vi "Fit Logistic Square Pulse.vi"(0 "Decay":T14, 1 "Optimal Offset Selection Criterion":T1, 5 "Boundaries":dbl[](array[numeric]), 9 "Basic Fit Options":T4, 11 "error in (no error)":errorcluster, 12 "Square Pulse Options":T2={"Method"=enum."Mode", "# Bins"=0, "Threshold %"=10.0, "Center on Midpoint"=TRUE, "Smoothen Plot"=FALSE}) -> (4 "Fitted Decay":cluster{"t Array":dbl[], "Fitted Array":dbl[]}, 6 "Residuals":cluster{"t Array":dbl[], "Residual Array":dbl[]}, 8 "Fit Output":T9={"best nonlinear fit"=[], "best fit parameters"=[], "R^2"=0.0, "RMSE"=0.0, "error out"={"status"=FALSE, "code"=0, "source"=""}, "Fitting Method"=enum."Least Square", "number of function calls"=0, "number of iterations"=0, "covariance"=[], "Chi 2"=0.0, "DOF"=0, "Fit Convergence Criterion"=enum."Continue", "Fitting Algorithm"=enum."Levenberg-Marquardt", "Weighted Fit"=enum."Unweighted", "Gradient"=0.0, "|Delta Chi 2|"=0.0, "|Delta Chi 2|/Chi 2"=0.0, "Max |Delta a| /|a|"=0.0, "Lambda"=-1.0, "RSS"=0.0, "AIC"=0.0, "BIC"=0.0, "Max number of function calls"=0, "Max number of iterations"=0, "IRF"={"X Array"=[], "Y Array"=[]}, "IRF Normalization Factor"=0.0, "Decay Normalization Factor"=0.0, "Number of offset fits"=0, "Weighted Chi2"=-1.0, "Unweighted Chi2"=-1.0}, 10 "Delta Best Fit Parameters":dbl[](array[numeric]), 15 "error out":errorcluster)   [LabVIEW 2021, in "Fits.lvlib"]
uses:
  Fits.lvlib
  ee5d1f48-236f-4ce4-8b82-c8db8954dd38.vi
  Time/Time.lvlib
  <vilib>/ErrorRing/Error Ring.xnode
  <vilib>/Utility/error.llb/DialogType.ctl
  LM model Function and gradient (Logistic Square-Gated IRF).vi
  <vilib>/Utility/error.llb/Error Cluster From Error Code.vi
  Arrays/Arrays.lvlib
  Graphs/XY Graph/XY Graph Plot Data.ctl
  Graphs/XY Graph/XY Graph Add-Ons.lvlib
  Decay Convolution/Fit Control Data.ctl
  <vilib>/Analysis/Matrix/Datatypes/RealMatrix.ctl
  <vilib>/Analysis/Matrix/NI_Matrix.lvlib
  Non-linear Fit Output v4.ctl
  Residual Type.ctl
  Basic Fit Options.ctl
  Square Pulse Levels Type.ctl
  Square Pulse Options.ctl
  Convergence Criteria.ctl
  Non-linear Fitting Algorithm.ctl
  Non-linear Fitting Method v2.ctl
  Nonlinear Fit Method.ctl
  Optimal Offset Selection Criterion.ctl
  IRF(X)PSED/Fit Weights Type v2.ctl
panel:
  out "XY Graph":cluster{"X Array":dbl[], "Y Array":dbl[]}[](graph)
  out "CPU (s)":dbl
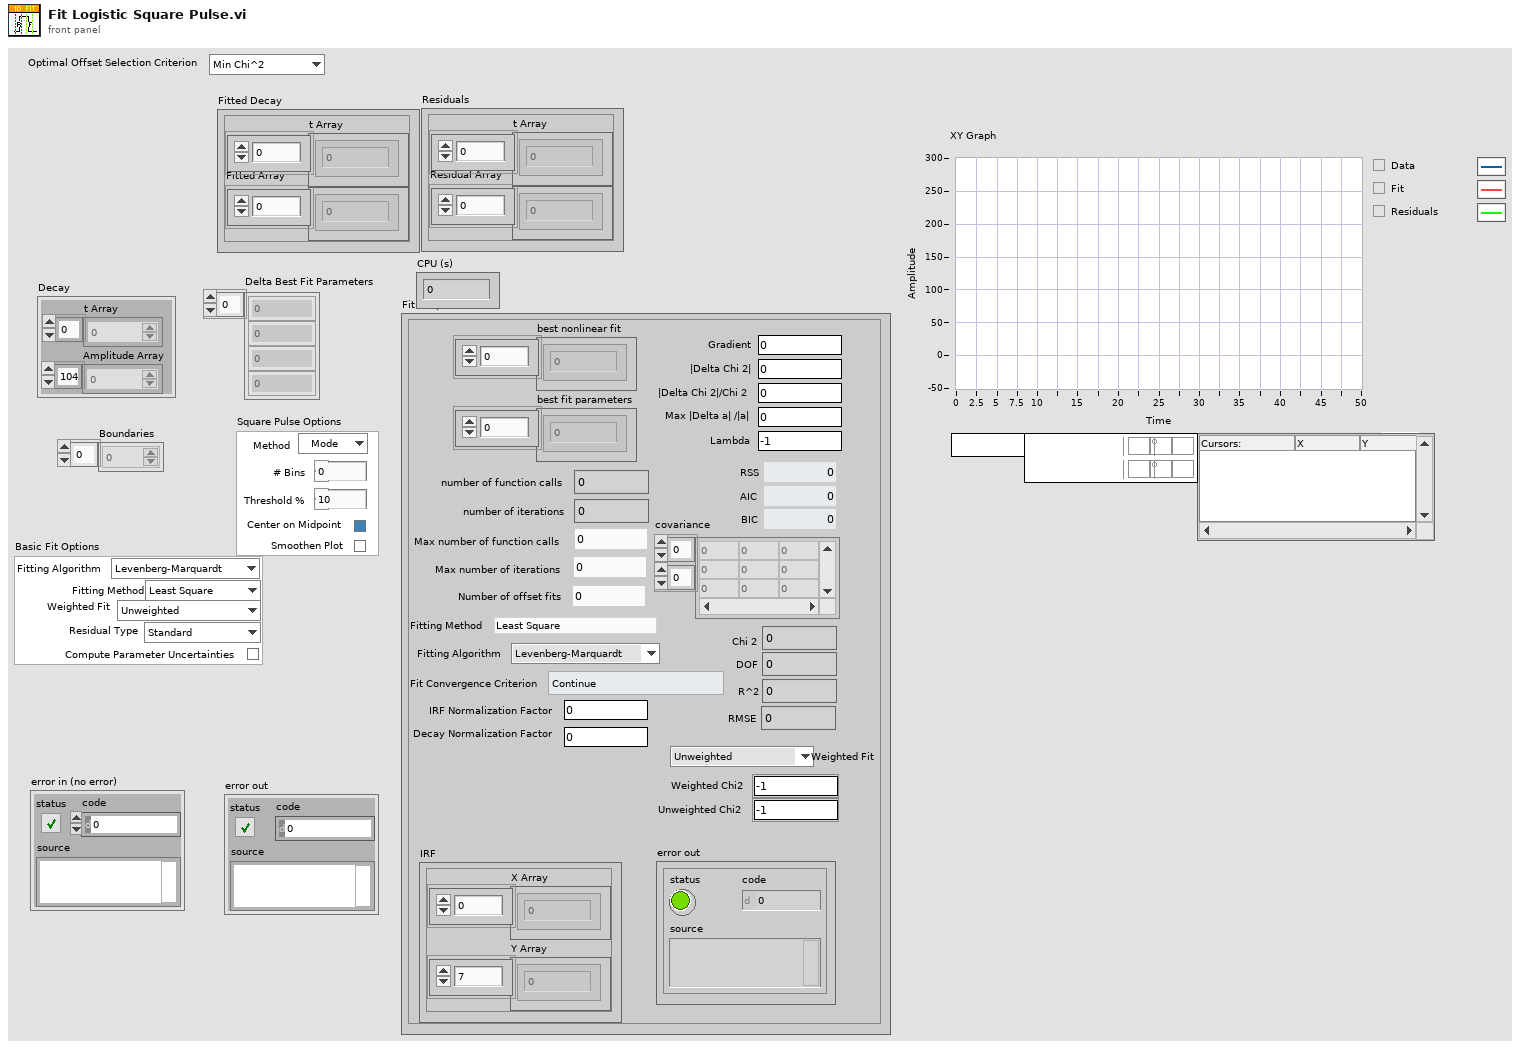
[diagram p1: front panel]
types:
  T1 = typedef "Fits.lvlib/Optimal Offset Selection Criterion.ctl" = enum16{"Min Chi^2", "Max R^2"}
  T2 = typedef "Fits.lvlib/Square Pulse Options.ctl" = cluster{"Method":T3, "# Bins":i32, "Threshold %":dbl, "Center on Midpoint":bool, "Smoothen Plot":bool}
  T3 = typedef "Fits.lvlib/Square Pulse Levels Type.ctl" = enum16{"Mode", "Mean"}
  T4 = typedef "Fits.lvlib/Basic Fit Options.ctl" = cluster{"Fitting Method":T5, "Weighted Fit":T6, "Residual Type":T7, "Compute Parameter Uncertainties":bool, "Fitting Algorithm":T8}
  T5 = typedef "Fits.lvlib/Non-linear Fitting Method v2.ctl" = enum16{"Least Square", "Least Absolute Residual", "Bisquare", "MLE", "-", "Best of All"}
  T6 = typedef "Fits.lvlib/Fit Weights Type v2.ctl" = enum16{"Unweighted", "1/Variance (Neyman)", "1/Variance (Pearson)", "Best of All"}
  T7 = typedef "Fits.lvlib/Residual Type.ctl" = enum16{"Standard", "Normalized", "Reduced"}
  T8 = typedef "Fits.lvlib/Non-linear Fitting Algorithm.ctl" = enum16{"Levenberg-Marquardt", "Trust-Region Dogleg"}
  T9 = typedef "Fits.lvlib/Non-linear Fit Output v4.ctl" = cluster{"best nonlinear fit":dbl[], "best fit parameters":dbl[], "R^2":dbl, "RMSE":dbl, "error out":errorcluster, "Fitting Method":T10, "number of function calls":i32, "number of iterations":i32, "covariance":T11, "Chi 2":dbl, "DOF":i32, "Fit Convergence Criterion":T12, "Fitting Algorithm":T8, "Weighted Fit":T6, "Gradient":dbl, "|Delta Chi 2|":dbl, "|Delta Chi 2|/Chi 2":dbl, "Max |Delta a| /|a|":dbl, "Lambda":dbl, "RSS":dbl, "AIC":dbl, "BIC":dbl, "Max number of function calls":i32, "Max number of iterations":i32, "IRF":T13, "IRF Normalization Factor":dbl, "Decay Normalization Factor":dbl, "Number of offset fits":i32, "Weighted Chi2":dbl, "Unweighted Chi2":dbl}
  T10 = typedef "Fits.lvlib/Nonlinear Fit Method.ctl" = enum16{"Least Square", "Least Absolute Residual", "Bisquare", "MLE"}
  T11 = typedef "NI_Matrix.lvlib/RealMatrix.ctl" = dbl[][]
  T12 = typedef "Fits.lvlib/Convergence Criteria.ctl" = enum16{"Continue", "Tolerances Exceeded", "Max Time Exceeded", "Max Iterations Exceeded", "Max Function Evaluations Exceeded", "Scale Range Exceeded"}
  T13 = typedef "XY Graph Add-Ons.lvlib/XY Graph Plot Data.ctl" = cluster{"X Array":dbl[], "Y Array":dbl[]}
  T14 = cluster{"t Array":dbl[], "Amplitude Array":dbl[]}
  T15 = cluster{"parameter minimum":dbl[], "parameter maximum":dbl[]}
  T16 = typedef "DialogType.ctl" = u16
  T17 = typedef "Fits.lvlib/Fit Control Data.ctl" = cluster{"IRF":T13, "Laser Period":dbl, "SYNC Period":dbl}
  T18 = cluster{"t Array":dbl[], "best nonlinear fit":dbl[]}
  T19 = cluster{"t Array":dbl[], "best nonlinear fit":dbl[]}[]
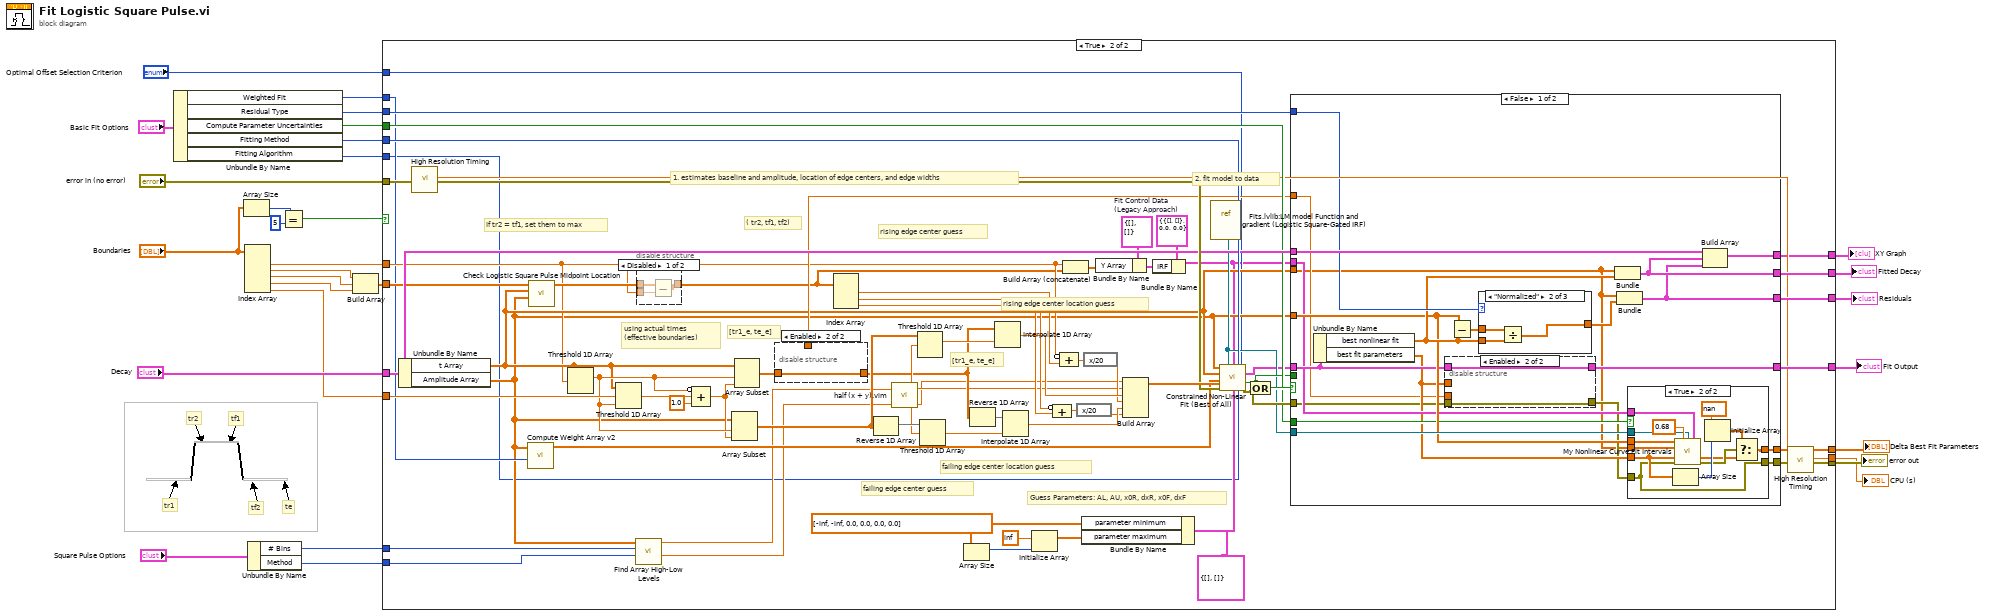
[diagram p0: block diagram]
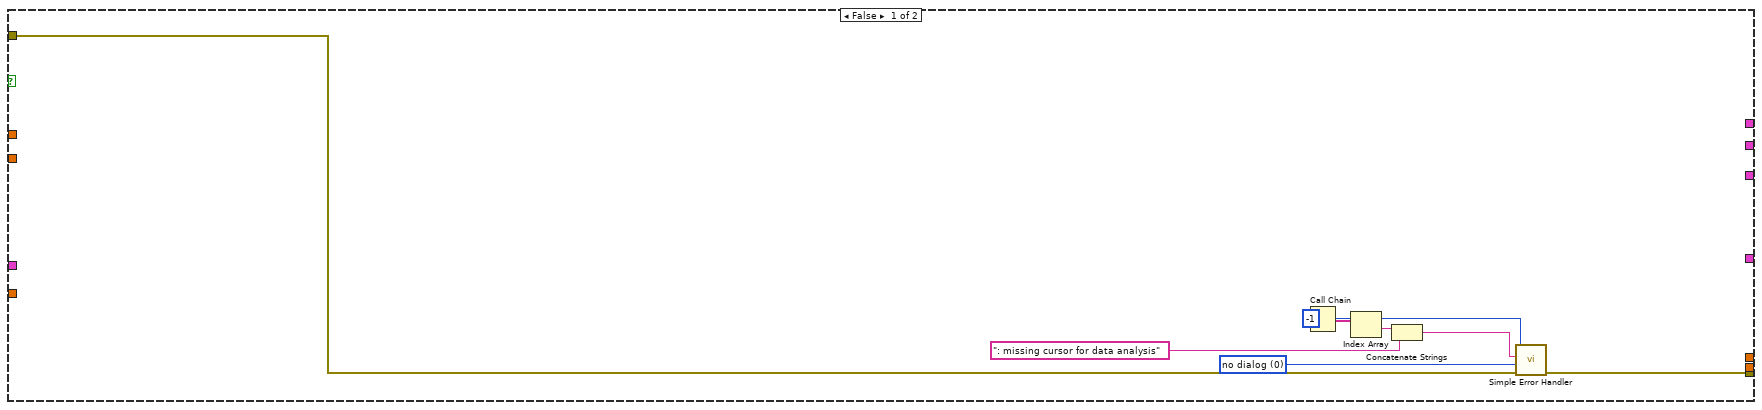
[diagram p2: hidden frame]
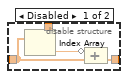
[diagram p4: hidden frame]
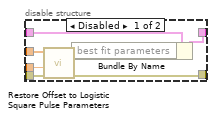
[diagram p5: hidden frame]
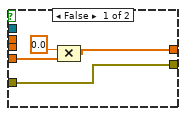
[diagram p6: hidden frame]
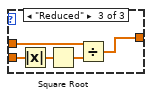
[diagram p8: hidden frame]
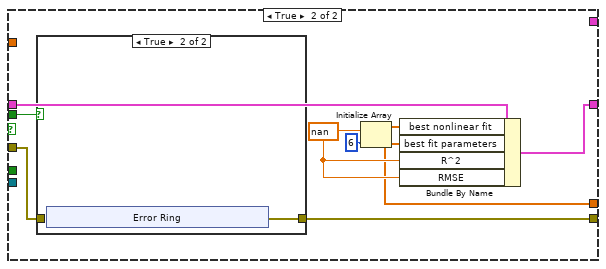
[diagram p9: hidden frame]
diagram:
  # "te"
  # "tf2"
  # "tf1"
  # "tr2"
  # "tr1"
  n1 = Unbundle By Name("Basic Fit Options") -> ("Weighted Fit"=w6:T6, "Residual Type"=w24:T7, "Compute Parameter Uncertainties"=w25:bool, "Fitting Method"=w27:T5, "Fitting Algorithm"=w2:T8)
  n2 = Array Size(array="Boundaries") -> (size(s)=w15:i32)
  n3 = Index Array(array="Boundaries") -> (element #1=w16:dbl, element #2=w10:dbl, element #3=w9:dbl, element #4=w13:dbl, element #5=w12:dbl)  [unwired: 5 in]
  n4 = Unbundle By Name("Square Pulse Options") -> ("# Bins"=w3:i32, "Method"=w4:T3)
  n5 = Equal?(x=w15, y=5) -> (x = y?=w11:bool)
  n6 = Build Array(w10, w9, w13) -> (w29:dbl[])
  n7 = case shown="True" w11 {
    tunnel: w29 -> [_ w64]
    tunnel: "error in (no error)" -> [w31 w98]
    tunnel: w27 -> [_ w97]
    tunnel: "Decay" -> [_ w87]
    tunnel: w25 -> [_ w86]
    tunnel: w24 -> [_ w85]
    tunnel: [_ w82] -> w23
    tunnel: [_ w81] -> w22
    tunnel: [_ w80] -> w21
    tunnel: [_ w79] -> w20
    tunnel: [w37 w78] -> w19
    tunnel: [_ w77] -> w18
    tunnel: [_ w75] -> w17
    tunnel: w16 -> [_ w54]
    tunnel: w12 -> [_ w74]
    tunnel: w6 -> [_ w53]
    tunnel: w4 -> [_ w49]
    tunnel: w3 -> [_ w48]
    tunnel: w2 -> [_ w46]
    tunnel: "Optimal Offset Selection Criterion" -> [_ w44]
    frame False {
      w36 = T16 0 items=["no dialog", "OK message", "continue or stop message", "OK message + warnings", "continue/stop + warnings"] ("type of dialog (OK msg:1)")
      n8 = Call Chain() -> (call chain=w35:string[])
      n9 = Index Array(array=w35) -> (element=w34:string)  [unwired: 1 in]
      n10 = Concatenate Strings(w34, ": missing cursor for data analysis" ("format string")) -> (w32:string)
      n11 = call <vilib>:"Simple Error Handler.vi"("error code (no error:0)"=-1, "error source (\" \")"=w32, "type of dialog (OK msg:1)"=w36, "error in (no error)"=w31) -> ("error out"=w37:errorcluster)  [unwired: 1 in, 4 out]
    }
    frame True {
      w43 = T17 {"IRF"={"X Array"=[], "Y Array"=[]}, "Laser Period"=0.0, "SYNC Period"=0.0}  # Fit Control Data (Legacy Approach)
      w67 = dbl[] [-inf, -inf, 0.0, 0.0, 0.0, 0.0] ("parameter minimum")
      # "2. fit model to data"
      # "1. estimates baseline and amplitude, location of edge centers, and edge widths"
      # "failing edge center location guess"
      # "failing edge center guess"
      # "rising edge center location guess"
      # "rising edge center guess"
      # "using actual times\n(effective boundaries)"
      # "If tr2 = tf1, set them to max"
      # "( tr2, tf1, tf2)"
      # "[tr1_e, te_e]"
      # "[tr1_e, te_e]"
      # "Guess Parameters: AL, AU, x0R, dxR, x0F, dxF"
      n12 = Unbundle By Name(w87) -> ("t Array"=w60:dbl[], "Amplitude Array"=w47:dbl[])
      n13 = call "High Resolution Timing.vi"("Error In"=w98) -> ("elapsed (relative) seconds"=w76:dbl, "Error Out"=w96:errorcluster)  [unwired: 16 in, 1 out]
      n14 = call "Compute Weight Array v2.vi"("Weighted Fit"=w53, "Data Array"=w47) -> ("Weight Array"=w52:dbl[])  [unwired: 8 in, 1 out]
      n15 = call "Check Logistic Square Pulse Midpoint Location.vi"("Amplitude Array"=w47, "t Array"=w60, "Cursors in"=w64) -> ("Cursors out"=w63:dbl[])  [unwired: 8 in]
      n16 = Threshold 1D Array(2:w54, 3:w60) -> (0:w72:dbl)  [unwired: 1 in]
      n17 = Threshold 1D Array(1:w72, 2:w74, 3:w60) -> (0:w73:dbl)
      n18 = call "Find Array High-Low Levels.vi"("Method (Mode)"=w49, "# Bins (auto)"=w48, "Array"=w47) -> ("Low Level"=w50:dbl, "High Level"=w51:dbl)  [unwired: 6 in, 1 out]
      n19 = disable-structure shown="Disabled" {
        disable-tunnel: [w109 w110] -> w39
        disable-tunnel: w54 -> [w108 _]
        disable-tunnel: w63 -> [w107 w110]
        frame Disabled {
          n20 = Subtract(x=w107, y=w108) -> (x-y=w109:dbl[])
        }
        frame Enabled {
        }
      }
      n21 = Compound Arithmetic op=ADD(invert w72, w73, 1.0 ("value")) -> (w70:dbl)
      n22 = Array Subset(array=w47, index=w72, length=w70) -> (w90:dbl[])
      n23 = Array Subset(array=w60, index=w72, length=w70) -> (w92:dbl[])
      n24 = disable-structure shown="Enabled" {
        disable-tunnel: w92 -> [w113 w114]
        disable-tunnel: [w112 w114] -> w89
        disable-tunnel: [w111 _] -> w61
        frame Disabled {
          n25 = Index Array(array=w113) -> (element=w111:dbl)  [unwired: 1 in]
          n26 = Compound Arithmetic op=ADD(invert w111, w113) -> (w112:dbl[])
        }
        frame Enabled {
        }
      }
      n27 = Index Array(array=w39) -> (element #1=w59:dbl, element #2=w55:dbl, element #3=w56:dbl)  [unwired: 3 in]
      n28 = Reverse 1D Array(array=w90) -> (reversed array=w104:dbl[])
      n29 = call "half (x + y).vim"("y"=w50, "x"=w51) -> ("(x+y)/2"=w103:dbl)  [unwired: 4 in]
      n30 = Threshold 1D Array(2:w103, 3:w90) -> (0:w105:dbl)  [unwired: 1 in]
      n31 = Threshold 1D Array(2:w103, 3:w104) -> (0:w102:dbl)  [unwired: 1 in]
      n32 = Array Size(array=w67) -> (size(s)=w66:i32)
      n33 = Reverse 1D Array(array=w89) -> (reversed array=w95:dbl[])
      n34 = Interpolate 1D Array(1:w105, 2:w89) -> (0:w100:dbl)
      n35 = Interpolate 1D Array(1:w102, 2:w95) -> (0:w101:dbl)
      n36 = Initialize Array(inf ("Numeric"), w66) -> (w65:dbl[])
      n37 = Compound Arithmetic op=ADD(invert w55, w56) -> (w57:dbl)
      n38 = Compound Arithmetic op=ADD(invert w54, w59) -> (w99:dbl)
      n39 = Build Array (concatenate)(w54, w39) -> (w40:dbl[])
      n40 = expression code="x/20"(w57) -> (w58:dbl)
      n41 = Bundle By Name(cluster=T15 {"parameter minimum"=[], "parameter maximum"=[]} ("parameter bounds"), "parameter minimum"=w67, "parameter maximum"=w65) -> (w94:T15)
      n42 = expression code="x/20"(w99) -> (w69:dbl)
      n43 = Bundle By Name(cluster=T13 {"X Array"=[], "Y Array"=[]} ("IRF"), "Y Array"=w40) -> (w41:T13)
      n44 = Build Array(w50, w51, w100, w69, w101, w58) -> (w106:dbl[])
      n45 = Bundle By Name(cluster=w43, "IRF"=w41) -> (w38:T17)
      n46 = vi-ref "Fits.lvlib:LM model Function and gradient (Logistic Square-Gated IRF).vi"() -> (w62:refnum<vi>)
      n47 = call "Constrained Non-Linear Fit (Best of All).vi"("Y Array"=w47, "f(x,a)"=w62, "Data"=w38, "Fitting Method"=w97, "Optimal Offset Selection Criterion"=w44, "X Array"=w60, "Weights"=w52, "Guess Fitted Parameters"=w106, "error in (no error)"=w96, "Fitted parameter bounds"=w94, "Fitting Algorithm"=w46) -> ("Fit Output"=w45:T9, "Fit Aborted?"=w84:bool, "Error Out"=w88:errorcluster)  [unwired: 1 in, 1 out]
      n48 = Compound Arithmetic op=OR(w84, w88) -> (w91:bool)
      n49 = case shown="False" w91 {
        tunnel: w87 -> [w135 _]
        tunnel: [w134 _] -> w75
        tunnel: [w133 _] -> w80
        tunnel: [w132 w176] -> w83
        tunnel: [w131 w172] -> w79
        tunnel: [w130 _] -> w81
        tunnel: w85 -> [w129 _]
        tunnel: w60 -> [w115 _]
        tunnel: w62 -> [w126 _]
        tunnel: w47 -> [w124 _]
        tunnel: w45 -> [w123 w175]
        tunnel: w88 -> [w119 w177]
        tunnel: [w117 w174] -> w82
        tunnel: w38 -> [w122 _]
        tunnel: w86 -> [w121 _]
        tunnel: w84 -> [_ w171]
        tunnel: w61 -> [w116 _]
        frame False {
          n50 = Unbundle By Name(w123) -> ("best nonlinear fit"=w125:dbl[], "best fit parameters"=w120:dbl[])
          n51 = disable-structure shown="Enabled" {
            disable-tunnel: w123 -> [w142 w144]
            disable-tunnel: w120 -> [w141 _]
            disable-tunnel: w119 -> [w140 w143]
            disable-tunnel: [w139 w143] -> w118
            disable-tunnel: [w138 w144] -> w117
            disable-tunnel: w116 -> [w136 _]
            frame Disabled {
              n52 = call "Restore Offset to Logistic Square Pulse Parameters.vi"("Error In"=w140, "Offset"=w136, "Best Fit Parameters"=w141) -> ("Error Out"=w139:errorcluster, "Offset Best Fit Parameters"=w137:dbl[])  [unwired: 7 in]
              n53 = Bundle By Name(cluster=w142, "best fit parameters"=w137) -> (w138:T9)
            }
            frame Enabled {
            }
          }
          n54 = Subtract(x=w124, y=w125) -> (x-y=w128:dbl[])
          n55 = case shown="\"Normalized\"" w129 {
            tunnel: w128 -> [w162 w165 w170]
            tunnel: [w162 w163 w168] -> w127
            tunnel: w125 -> [_ w164 w169]
            frame "Standard", Default {
            }
            frame "Normalized" {
              n56 = Divide(x=w165, y=w164) -> (x/y=w163:dbl[])
            }
            frame "Reduced" {
              n57 = Absolute Value(x=w169) -> (abs(x)=w167:dbl[])
              n58 = Square Root(x=w167) -> (sqrt(x)=w166:dbl[])
              n59 = Divide(x=w170, y=w166) -> (x/y=w168:dbl[])
            }
          }
          n60 = Bundle("t Array"=w115, "best nonlinear fit"=w125) -> (w133:T18)  [unwired: 1 in]
          n61 = Bundle("t Array"=w115, w127) -> (w130:cluster{"t Array":dbl[], dbl[]})  [unwired: 1 in]
          n62 = case shown="True" w121 {
            tunnel: [w148 w149] -> w132
            tunnel: [w146 w150] -> w131
            tunnel: w115 -> [_ w160]
            tunnel: w126 -> [_ w159]
            tunnel: w122 -> [_ w158]
            tunnel: w120 -> [w147 w156]
            tunnel: w124 -> [_ w157]
            tunnel: w118 -> [w148 w149]
            frame False {
              n63 = Compound Arithmetic op=MULTIPLY(0.0, w147) -> (w146:dbl[])
            }
            frame True {
              n64 = Array Size(array=w156) -> (size(s)=w155:i32)
              n65 = call "My Nonlinear Curve Fit Intervals.vi"("Y"=w157, "confidence level"=0.68, "f(x,a)"=w159, "data"=w158, "X"=w160, "best fit parameters"=w156, "error in (no error)"=w149) -> ("delta best fit parameters"=w151:dbl[], "error out"=w152:errorcluster)  [unwired: 7 in]
              n66 = Initialize Array(nan ("element"), w155) -> (w153:dbl[])
              n67 = Select(t=w153, s=w152, f=w151) -> (s? t:f=w150:dbl[])
            }
          }
          n68 = Build Array(w135, w133, w130) -> (w134:T19)
        }
        frame True {
          w173 = nan ("element")
          n69 = case shown="False" w171 {
            tunnel: w177 -> [w179 _]
            tunnel: [w179 w180] -> w176
            frame False {
            }
            frame True {
              n70 = xnode "Error Ring"() -> ("error out"=w180:errorcluster)
            }
          }
          n71 = Initialize Array(w173, 6 ("dimension size")) -> (w172:dbl[])
          n72 = Bundle By Name(cluster=w175, "best nonlinear fit"=w172, "best fit parameters"=w172, "R^2"=w173, "RMSE"=w173) -> (w174:T9)
        }
      }
      n73 = call "High Resolution Timing.vi"("relative seconds (NaN)"=w76, "Error In"=w83) -> ("elapsed (relative) seconds"=w77:dbl, "Error Out"=w78:errorcluster)  [unwired: 15 in, 1 out]
    }
  }
  "error out" <- w19
  "Fit Output" <- w23
  "Residuals" <- w22
  "Fitted Decay" <- w21
  "Delta Best Fit Parameters" <- w20
  "CPU (s)" <- w18
  "XY Graph" <- w17
